vi "Read ECU Software ID.vi"(6 "error in":errorcluster, 8 "MaxRead":i32, 9 "Channel in":u16) -> (0 "error out":errorcluster, 1 "Messages":T1(array[cluster]), 2 "Pass":bool, 3 "Channel out":u16, 4 "ECU Software ID":string)   [LabVIEW 2023]
uses:
  041652ea-0565-4739-b3a0-c3d9c3bdead1.vi
  83aec2fd-9d4c-4c8f-91a5-b1bc64c9b534.vi
  4f930f32-d09a-43ef-bca1-8b214b378bd5.vi
  9d70b389-ba7c-43d5-b065-c738d8b1377d.vi
  85706bb4-c733-458b-aff3-8e9b4f8b92f2.vi
  939cf2b4-caa2-4f33-bd1d-4e781c063efc.vi
  e8470de1-fa2d-4ee3-b50e-96bd89dc731f.vi
  d0f02419-cfb7-4a5e-bc3c-f035efdb0e96.vi
  Communication/PCAN2023/PCAN API.lvlib
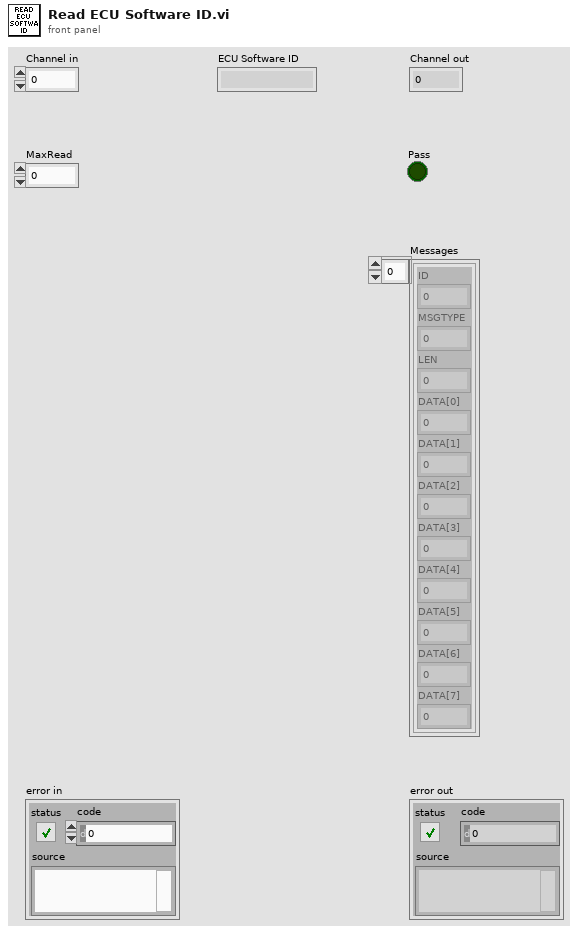
[diagram p1: front panel]
types:
  T1 = cluster{"ID":u32, "MSGTYPE":u8, "LEN":u8, "DATA[0]":u8, "DATA[1]":u8, "DATA[2]":u8, "DATA[3]":u8, "DATA[4]":u8, "DATA[5]":u8, "DATA[6]":u8, "DATA[7]":u8}[]
  T2 = cluster{"ID":u32, "MSGTYPE":u8, "LEN":u8, "DATA[0]":u8, "DATA[1]":u8, "DATA[2]":u8, "DATA[3]":u8, "DATA[4]":u8, "DATA[5]":u8, "DATA[6]":u8, "DATA[7]":u8}
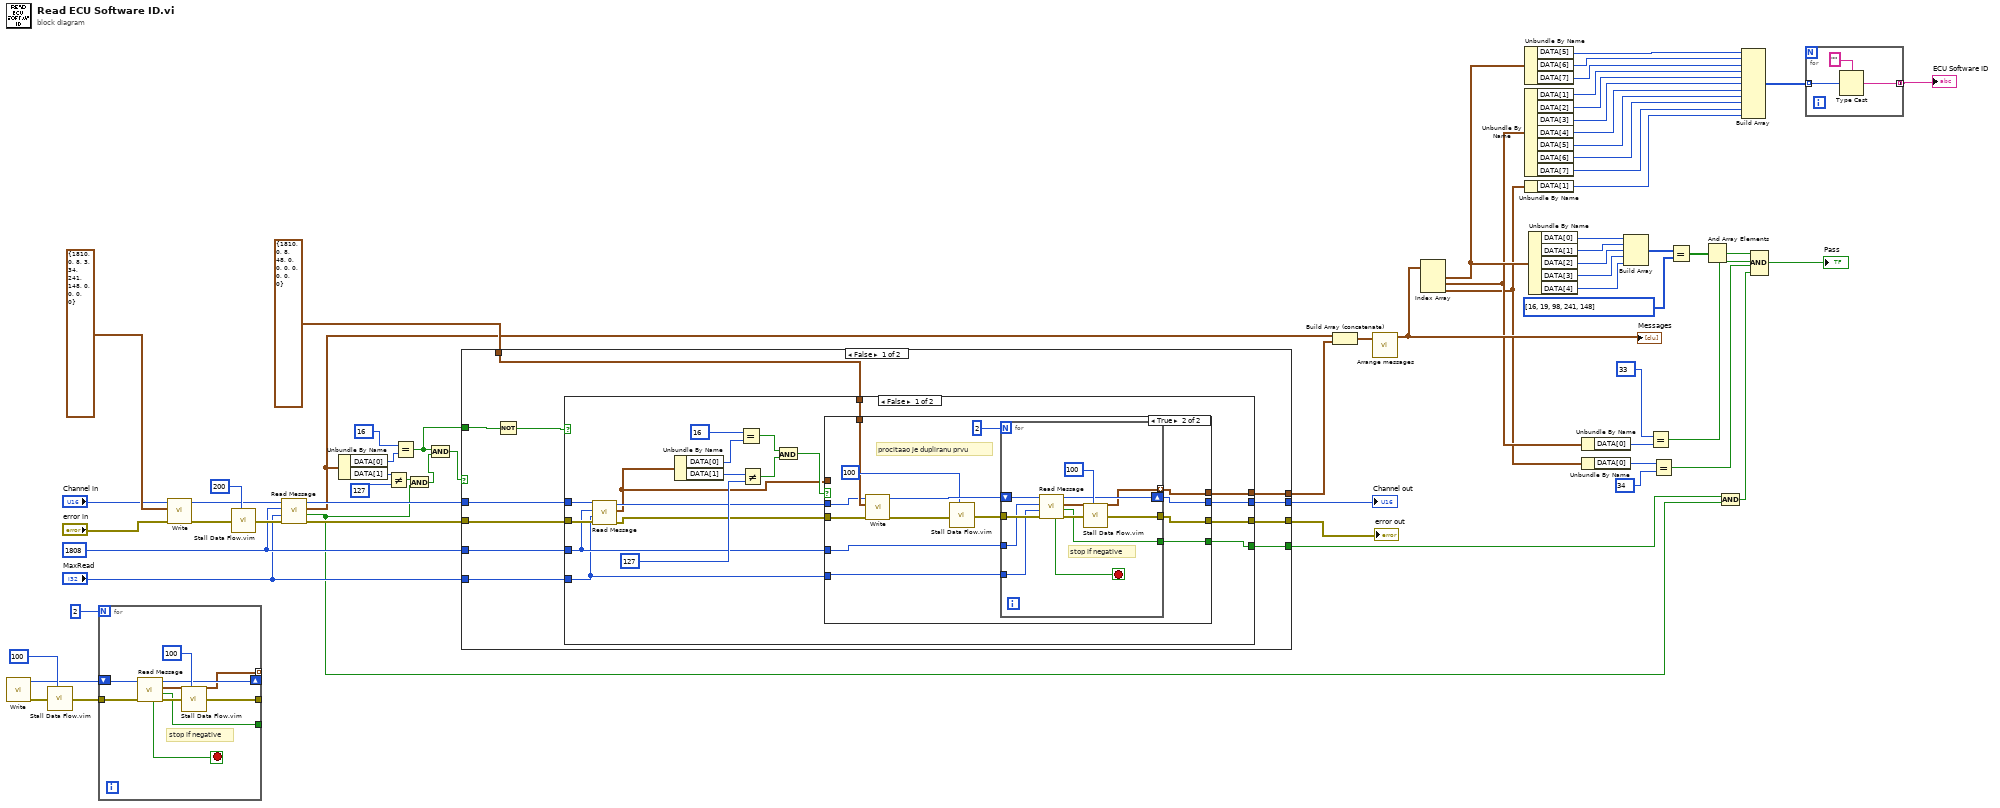
[diagram p0: block diagram]
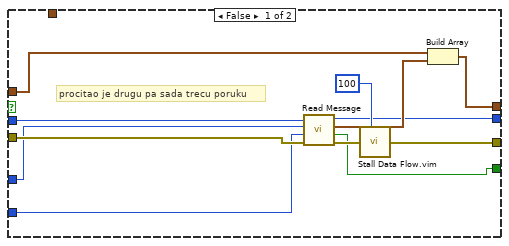
[diagram p2: hidden frame]
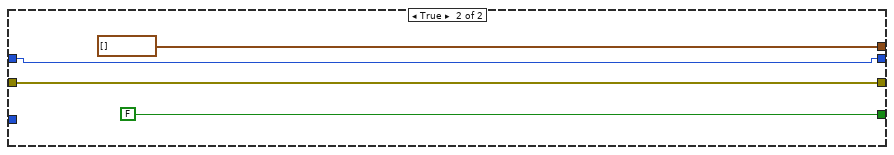
[diagram p3: hidden frame]
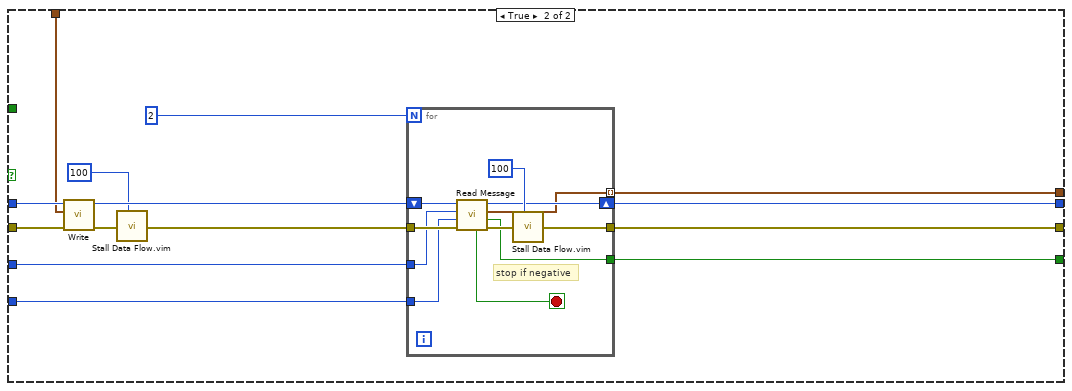
[diagram p4: hidden frame]
diagram:
  (unwired) u32 200 ("milliseconds to wait")
  w19 = u32 1808 ("ID")
  n1 = call "Write.vi"() -> ("error out"=w10:errorcluster, "Channel out"=w6:u16)  [unwired: 8 in, 2 out]
  n2 = call "Stall Data Flow.vim"("value in"=w10, "milliseconds to wait"=u32 100) -> ("value out"=w7:errorcluster)  [unwired: 1 out]
  n3 = for {
    N: 2 -> [_]
    tunnel: [w68] -> _
    shift-right: [w72] -> _
    shift-left: w6 -> [w73]
    tunnel: w7 -> [w71]
    tunnel: [w75] -> _
    tunnel: [w69] -> _ mode=indexing
    stop <- w67 stop-if-true
    # "stop if negative"
    n4 = call "Read Message.vi"("error in"=w71, "Channel in"=w73) -> ("error out"=w70:errorcluster, "Passed"=w68:bool, "Last Message"=w69:T2, "Channel out"=w72:u16, "Negative"=w67:bool)  [unwired: 5 in]
    n5 = call "Stall Data Flow.vim"("value in"=w70, "milliseconds to wait"=u32 100) -> ("value out"=w75:errorcluster)  [unwired: 1 out]
  }
  n6 = call "Write.vi"("error in"="error in", "MessageBuffer"=T2 {"ID"=1810, "MSGTYPE"=0, "LEN"=8, "DATA[0]"=3, "DATA[1]"=34, "DATA[2]"=241, "DATA[3]"=148, "DATA[4]"=0, "DATA[5]"=0, "DATA[6]"=0, "DATA[7]"=0}, "Channel"="Channel in") -> ("error out"=w62:errorcluster, "Channel out"=w24:u16)  [unwired: 5 in, 2 out]
  n7 = call "Stall Data Flow.vim"("value in"=w62, "milliseconds to wait"=u32 200) -> ("value out"=w22:errorcluster)  [unwired: 1 out]
  n8 = call "Read Message.vi"("error in"=w22, "MaxRead"="MaxRead", "ID"=w19, "Channel in"=w24) -> ("error out"=w21:errorcluster, "Passed"=w16:bool, "Last Message"=w20:T2, "Channel out"=w23:u16)  [unwired: 3 in, 1 out]
  n9 = Unbundle By Name(w20) -> ("DATA[0]"=w14:u8, "DATA[1]"=w57:u8)
  n10 = Not Equal?(x=w57, y=u8 127) -> (x != y?=w17:bool)
  n11 = Equal?(x=u8 16 ("y"), y=w14) -> (x = y?=w11:bool)
  n12 = And(x=w17, y=w16) -> (x .and. y?=w13:bool)
  n13 = And(x=w11, y=w13) -> (x .and. y?=w12:bool)
  n14 = case shown="False" w12 {
    tunnel: w23 -> [w82 w160]
    tunnel: w21 -> [w81 w159]
    tunnel: [w76 w158] -> w61
    tunnel: [w85 w157] -> w60
    tunnel: [w77 w155] -> w59
    tunnel: T2 {"ID"=1810, "MSGTYPE"=0, "LEN"=8, "DATA[0]"=48, "DATA[1]"=0, "DATA[2]"=0, "DATA[3]"=0, "DATA[4]"=0, "DATA[5]"=0, "DATA[6]"=0, "DATA[7]"=0} ("MessageBuffer") -> [w78 w153]
    tunnel: [w86 w149] -> w30
    tunnel: w19 -> [w80 w148]
    tunnel: "MaxRead" -> [w79 w147]
    tunnel: w11 -> [w84 _]
    frame False {
      n15 = Not(x=w84) -> (.not. x?=w83:bool)
      n16 = case shown="False" w83 {
        tunnel: [w88 T1 []] -> w86
        tunnel: [w96 FALSE] -> w85
        tunnel: w82 -> [w105 w144]
        tunnel: w81 -> [w104 w143]
        tunnel: w80 -> [w94 _]
        tunnel: w79 -> [w93 _]
        tunnel: w78 -> [w95 _]
        tunnel: [w90 w144] -> w77
        tunnel: [w89 w143] -> w76
        frame False {
          n17 = call "Read Message.vi"("error in"=w104, "MaxRead"=w93, "ID"=w94, "Channel in"=w105) -> ("error out"=w91:errorcluster, "Last Message"=w87:T2, "Channel out"=w92:u16)  [unwired: 3 in, 2 out]
          n18 = Unbundle By Name(w87) -> ("DATA[0]"=w103:u8, "DATA[1]"=w101:u8)
          n19 = Equal?(x=u8 16 ("y"), y=w103) -> (x = y?=w99:bool)
          n20 = Not Equal?(x=w101, y=u8 127) -> (x != y?=w98:bool)
          n21 = And(x=w99, y=w98) -> (x .and. y?=w97:bool)
          n22 = case shown="True" w97 {
            tunnel: [w110 w126] -> w96
            tunnel: w95 -> [_ w125]
            tunnel: w94 -> [w107 w124]
            tunnel: w93 -> [w106 w123]
            tunnel: w92 -> [w109 w122]
            tunnel: w91 -> [w108 w121]
            tunnel: [w112 w120] -> w90
            tunnel: [w111 w119] -> w89
            tunnel: [w117 w118] -> w88
            tunnel: w87 -> [w114 _]
            frame False {
              # "procitao je drugu pa sada trecu poruku"
              n23 = call "Read Message.vi"("error in"=w108, "MaxRead"=w106, "ID"=w107, "Channel in"=w109) -> ("error out"=w115:errorcluster, "Passed"=w110:bool, "Last Message"=w113:T2, "Channel out"=w112:u16)  [unwired: 3 in, 1 out]
              n24 = call "Stall Data Flow.vim"("value in"=w115, "milliseconds to wait"=u32 100) -> ("value out"=w111:errorcluster)  [unwired: 1 out]
              n25 = Build Array(w114, w113) -> (w117:T1)
            }
            frame True {
              # "procitaao je dupliranu prvu"
              n26 = call "Write.vi"("error in"=w121, "MessageBuffer"=w125, "Channel"=w122) -> ("error out"=w127:errorcluster, "Channel out"=w131:u16)  [unwired: 5 in, 2 out]
              n27 = call "Stall Data Flow.vim"("value in"=w127, "milliseconds to wait"=u32 100) -> ("value out"=w130:errorcluster)  [unwired: 1 out]
              n28 = for {
                N: 2 -> [_]
                tunnel: [w135] -> w126
                shift-right: [w139] -> w120
                shift-left: w131 -> [w140]
                tunnel: w130 -> [w138]
                tunnel: [w142] -> w119
                tunnel: [w136] -> w118 mode=indexing
                tunnel: w124 -> [w133]
                tunnel: w123 -> [w132]
                stop <- w134 stop-if-true
                # "stop if negative"
                n29 = call "Read Message.vi"("error in"=w138, "MaxRead"=w132, "ID"=w133, "Channel in"=w140) -> ("error out"=w137:errorcluster, "Passed"=w135:bool, "Last Message"=w136:T2, "Channel out"=w139:u16, "Negative"=w134:bool)  [unwired: 3 in]
                n30 = call "Stall Data Flow.vim"("value in"=w137, "milliseconds to wait"=u32 100) -> ("value out"=w142:errorcluster)  [unwired: 1 out]
              }
            }
          }
        }
        frame True {
        }
      }
    }
    frame True {
      n31 = call "Write.vi"("error in"=w159, "MessageBuffer"=w153, "Channel"=w160) -> ("error out"=w150:errorcluster, "Channel out"=w156:u16)  [unwired: 5 in, 2 out]
      n32 = call "Stall Data Flow.vim"("value in"=w150, "milliseconds to wait"=u32 100) -> ("value out"=w154:errorcluster)  [unwired: 1 out]
      n33 = for {
        N: 2 -> [_]
        tunnel: [w164] -> w157
        shift-right: [w168] -> w155
        shift-left: w156 -> [w169]
        tunnel: w154 -> [w167]
        tunnel: [w171] -> w158
        tunnel: [w165] -> w149 mode=indexing
        tunnel: w148 -> [w162]
        tunnel: w147 -> [w161]
        stop <- w163 stop-if-true
        # "stop if negative"
        n34 = call "Read Message.vi"("error in"=w167, "MaxRead"=w161, "ID"=w162, "Channel in"=w169) -> ("error out"=w166:errorcluster, "Passed"=w164:bool, "Last Message"=w165:T2, "Channel out"=w168:u16, "Negative"=w163:bool)  [unwired: 3 in]
        n35 = call "Stall Data Flow.vim"("value in"=w166, "milliseconds to wait"=u32 100) -> ("value out"=w171:errorcluster)  [unwired: 1 out]
      }
    }
  }
  "error out" <- w61
  "Channel out" <- w59
  n36 = Build Array (concatenate)(w20, w30) -> (w5:T1)
  n37 = call "Arrange messages.vi"("Array in"=w5) -> ("Array out"=w4:T1)  [unwired: 10 in]
  "Messages" <- w4
  n38 = Index Array(array=w4) -> (element #1=w3:T2, element #2=w2:T2, element #3=w1:T2)  [unwired: 3 in]
  n39 = Unbundle By Name(w3) -> ("DATA[5]"=w40:u8, "DATA[6]"=w39:u8, "DATA[7]"=w38:u8)
  n40 = Unbundle By Name(w2) -> ("DATA[1]"=w35:u8, "DATA[2]"=w34:u8, "DATA[3]"=w33:u8, "DATA[4]"=w32:u8, "DATA[5]"=w31:u8, "DATA[6]"=w27:u8, "DATA[7]"=w26:u8)
  n41 = Unbundle By Name(w1) -> ("DATA[1]"=w25:u8)
  n42 = Unbundle By Name(w3) -> ("DATA[0]"=w55:u8, "DATA[1]"=w54:u8, "DATA[2]"=w53:u8, "DATA[3]"=w52:u8, "DATA[4]"=w51:u8)
  n43 = Unbundle By Name(w2) -> ("DATA[0]"=w48:u8)
  n44 = Unbundle By Name(w1) -> ("DATA[0]"=w45:u8)
  n45 = Build Array(w55, w54, w53, w52, w51) -> (w50:u8[])
  n46 = Equal?(x=u8 33, y=w48) -> (x = y?=w43:bool)
  n47 = Equal?(x=w45, y=u8 34 ("x")) -> (x = y?=w41:bool)
  n48 = Equal?(x=w50, y=u8[] [16, 19, 98, 241, 148]) -> (x = y?=w44:bool[])
  n49 = And Array Elements(Boolean array=w44) -> (logical AND=w42:bool)
  n50 = Compound Arithmetic op=AND(w60, w16) -> (w28:bool)
  n51 = Build Array(w40, w39, w38, w35, w34, w33, w32, w31, w27, w26, w25) -> (w37:u8[])
  n52 = Compound Arithmetic op=AND(w42, w43, w41, w28) -> (→"Pass":bool)
  n53 = for {
    tunnel: w37 -> [w173] mode=indexing
    tunnel: [w172] -> w36 mode=concatenating
    n54 = Type Cast(type="", x=w173) -> (*(type *) &x=w172:string)
  }
  "ECU Software ID" <- w36
